vi "_attribute_read_boolean.vi"(5 "Repeated Capability":string, 7 "Attribute":T1={"Identifier"="", "Descriptive Name"="", "Data Type"=enum."Integer 32", "Command"="", "Access"=enum."Read/Write", "Range Table"="", "Read Callback"="", "Write Callback"="", "Supported Models"="", "Instrument Options"="", "Index"=0, "OPC Wait"=FALSE, "No Status Check"=FALSE, "Cache Only"=FALSE}, 8 "error in":errorcluster caption="error in (no error)", 10 "Query Parameter":string, 11 "VISA resource name":refnum<visa-resource-name>) -> (0 "error out":errorcluster, 2 "Boolean out":bool, 3 "VISA resource name out":refnum<visa-resource-name>)   [LabVIEW 2022 SP3, in "hmp4000_rsidr_core.lvlib"]
uses:
  hmp4000_rsidr_core.lvlib
  type_Attribute.ctl
  type_Attribute_Data_Type.ctl
  type_ReadWriteAccess.ctl
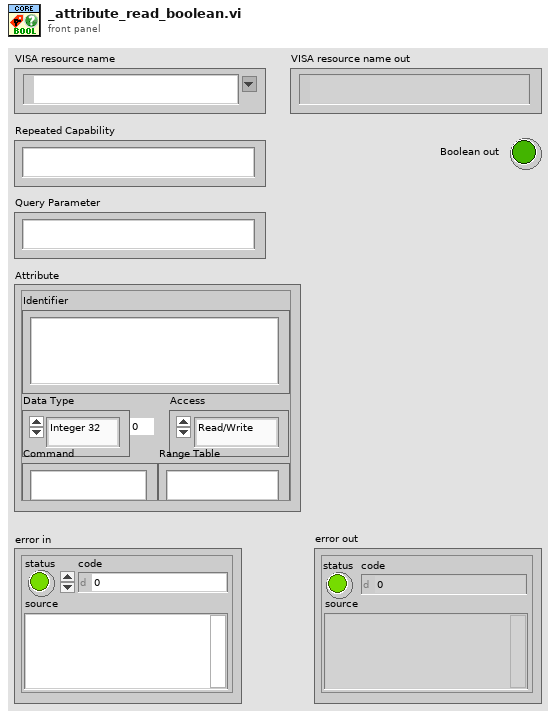
[diagram p1: front panel]
types:
  T1 = typedef "hmp4000_rsidr_core.lvlib/type_Attribute.ctl" = cluster{"Identifier":string, "Descriptive Name":string, "Data Type":T2, "Command":string, "Access":T3, "Range Table":string, "Read Callback":string, "Write Callback":string, "Supported Models":string, "Instrument Options":string, "Index":i32, "OPC Wait":bool, "No Status Check":bool, "Cache Only":bool}
  T2 = typedef "hmp4000_rsidr_core.lvlib/type_Attribute_Data_Type.ctl" = enum16{"Integer 32", "Double", "String", "Boolean", "None", "Integer 64", "RawString"}
  T3 = typedef "hmp4000_rsidr_core.lvlib/type_ReadWriteAccess.ctl" = enum16{"Read Only", "Write Only", "Read/Write"}
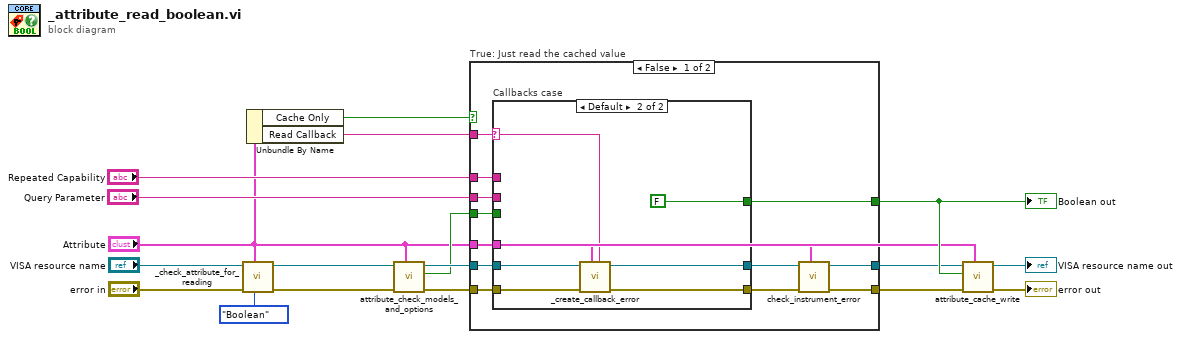
[diagram p0: block diagram]
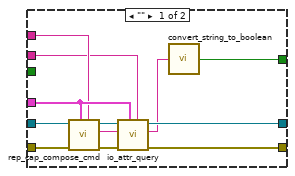
[diagram p2: hidden frame]
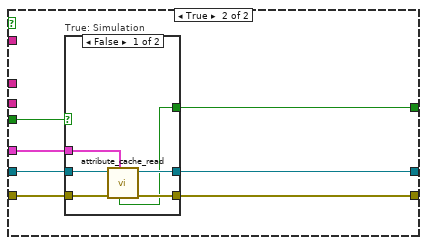
[diagram p3: hidden frame]
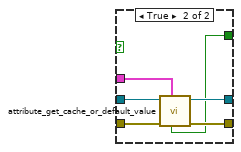
[diagram p4: hidden frame]
diagram:
  n1 = call "_check_attribute_for_reading.vi"("Expected Data Type"=type_Attribute_Data_Type."Boolean" ("Data Type"), "Attribute"="Attribute", "error in"="error in", "VISA resource name"="VISA resource name") -> ("error out"=w9:errorcluster, "VISA resource name out"=w8:refnum<visa-resource-name>)  [unwired: 6 in]
  n2 = Unbundle By Name("Attribute") -> ("Cache Only"=w1:bool, "Read Callback"=w10:string)
  n3 = call "attribute_check_models_and_options.vi"("Attribute"="Attribute", "error in"=w9, "VISA resource name"=w8) -> ("error out"=w7:errorcluster, "Simulation Mode"=w5:bool, "VISA resource name out"=w6:refnum<visa-resource-name>)  [unwired: 6 in]
  n4 = case "True: Just read the cached value" shown="False" w1 {
    tunnel: "Repeated Capability" -> [w30 _]
    tunnel: [w21 w53] -> w4
    tunnel: [w29 w50] -> w15
    tunnel: w10 -> [w28 _]
    tunnel: w6 -> [w27 w56]
    tunnel: w7 -> [w26 w55]
    tunnel: "Attribute" -> [w19 w51]
    tunnel: w5 -> [w25 w52]
    tunnel: [w20 w54] -> w3
    tunnel: "Query Parameter" -> [w24 _]
    frame False {
      n5 = case "Callbacks case" shown="Default" w28 {
        selector: w28 -> [_ w44]
        tunnel: w27 -> [w42 w48]
        tunnel: w26 -> [w41 w49]
        tunnel: w30 -> [w35 _]
        tunnel: [w40 w46] -> w22
        tunnel: [w34 w47] -> w23
        tunnel: [w33 FALSE ("Attribute Value Boolean")] -> w29
        tunnel: w19 -> [w36 w45]
        tunnel: w25 -> [_ _]
        tunnel: w24 -> [w31 _]
        frame "" {
          n6 = call "rep_cap_compose_cmd.vi"("Repeated Capability"=w35, "Attribute"=w36, "error in"=w41, "VISA resource name"=w42) -> ("error out"=w39:errorcluster, "Command out"=w38:string, "VISA resource name out"=w37:refnum<visa-resource-name>)  [unwired: 5 in]
          n7 = call "io_attr_query.vi"("Query Parameter (None)"=w31, "Attribute"=w36, "error in"=w39, "write buffer"=w38, "VISA resource name"=w37) -> ("error out"=w34:errorcluster, "read buffer"=w32:string, "VISA resource name out"=w40:refnum<visa-resource-name>)  [unwired: 4 in]
          n8 = call "convert_string_to_boolean.vi"("String in"=w32) -> ("boolean value out"=w33:bool)  [unwired: 4 in]
        }
        frame Default {
          n9 = call "_create_callback_error.vi"("Callback Name"=w44, "Attribute"=w45, "error in"=w49, "VISA resource name"=w48) -> ("error out"=w47:errorcluster, "VISA resource name out"=w46:refnum<visa-resource-name>)  [unwired: 6 in]
        }
      }
      n10 = call "check_instrument_error.vi"("Attribute"=w19, "error in"=w23, "VISA resource name"=w22) -> ("error out"=w21:errorcluster, "VISA resource name out"=w20:refnum<visa-resource-name>)  [unwired: 7 in]
    }
    frame True {
      n11 = case "True: Simulation" shown="False" w52 {
        tunnel: w55 -> [w62 w68]
        tunnel: w56 -> [w61 w67]
        tunnel: w51 -> [w60 w64]
        tunnel: [w59 w66] -> w53
        tunnel: [w58 w65] -> w54
        tunnel: [w57 w63] -> w50
        frame False {
          n12 = call "attribute_cache_read.vi"("Attribute"=w60, "error in"=w62, "VISA resource name"=w61) -> ("error out"=w59:errorcluster, "VISA resource name out"=w58:refnum<visa-resource-name>, "Boolean out"=w57:bool)  [unwired: 1 in, 5 out]
        }
        frame True {
          n13 = call "attribute_get_cache_or_default_value.vi"("Attribute"=w64, "error in"=w68, "VISA resource name"=w67) -> ("error out"=w66:errorcluster, "VISA resource name out"=w65:refnum<visa-resource-name>, "Boolean out"=w63:bool)  [unwired: 1 in, 5 out]
        }
      }
    }
  }
  "Boolean out" <- w15
  n14 = call "attribute_cache_write.vi"("Attribute"="Attribute", "error in"=w4, "Value in"=w15, "VISA resource name"=w3) -> ("error out"=→"error out":errorcluster, "VISA resource name out"=→"VISA resource name out":refnum<visa-resource-name>)  [unwired: 6 in]
